vi "TempEinzelmessungSub.vi"(2 "error in":errorcluster, 3 "mode (0)":i16, 4 "address string":string) -> (0 "error out":errorcluster, 1 "Numeric":dbl)   [LabVIEW 2010]
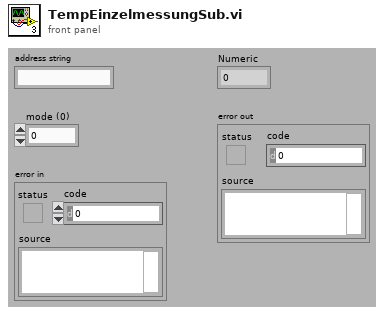
[diagram p1: front panel]
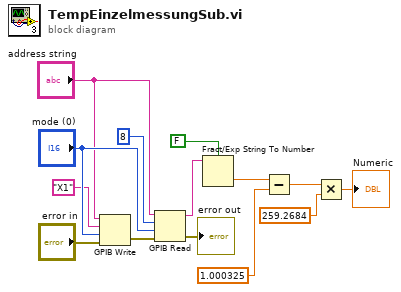
[diagram p0: block diagram]
diagram:
  n1 = GPIB Write(0:"address string", 1:"X1", 2:"mode (0)", 3:"error in") -> (6:w2:errorcluster)  [unwired: 1 in, 1 out]
  n2 = GPIB Read(0:"address string", 1:8, 2:"mode (0)", 3:w2) -> (5:w6:string, 7:→"error out":errorcluster)  [unwired: 1 in, 1 out]
  n3 = Fract/Exp String To Number(use system decimal point (T)=FALSE, string=w6) -> (number=w7:dbl)  [unwired: 2 in, 1 out]
  n4 = Subtract(x=w7, y=1.000325) -> (x-y=w8:dbl)
  n5 = Multiply(x=w8, y=259.2684) -> (x*y=→"Numeric":dbl)
